vi "testconandread.vi"() -> ()   [LabVIEW 2018]
panel:
  out "read buffer":string
  out "error out":errorcluster
  out "VISA resource name out":refnum<visa-resource-name>
  in  "baud rate (9600)":u32=9600
  in  "VISA resource name":refnum<visa-resource-name>
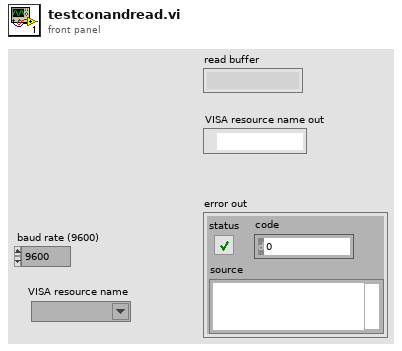
[diagram p1: front panel]
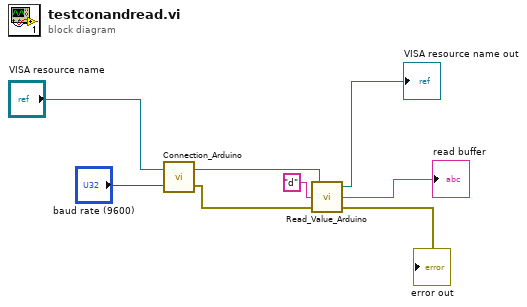
[diagram p0: block diagram]
diagram:
  n1 = call "Connection_Arduino.vi"("baud rate (9600)"="baud rate (9600)", "VISA resource name"="VISA resource name") -> ("error out"=w5:errorcluster, "VISA resource name out"=w6:refnum<visa-resource-name>)
  n2 = call "Read_Value_Arduino.vi"("error in (no error)"=w5, "write buffer"="d", "VISA resource name"=w6) -> ("error out"=→"error out":errorcluster, "read buffer"=→"read buffer":string, "VISA resource name out"=→"VISA resource name out":refnum<visa-resource-name>)
